vi "Create.vi"(8 "error in (no error)":errorcluster, 11 "ClientApp1 in":refnum<class "ClientApp1.lvclass">) -> (0 "error out":errorcluster, 3 "ClientApp1 out":refnum<class "ClientApp1.lvclass">)   [LabVIEW 2020, in "ClientApp1Lib.lvlib" / "ClientApp1.lvclass"]
uses:
  ClientApp1.lvclass
  C:/Users/dzoni/Documents/NJ/Playground/LV/Remote/ClientBase/ClientBase.lvclass
  ClientBase/ClientBase.lvclass
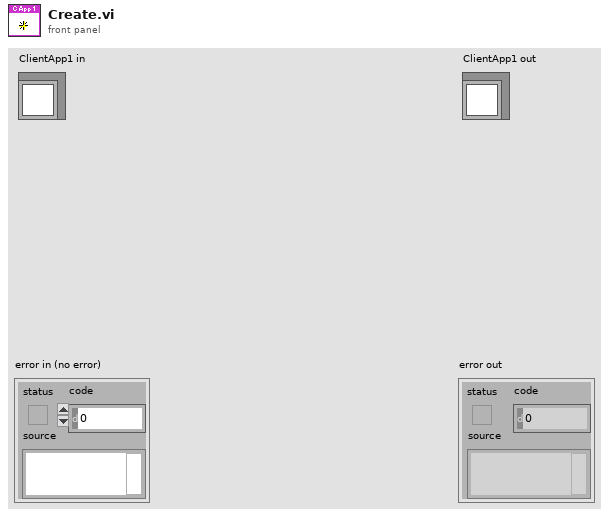
[diagram p1: front panel]
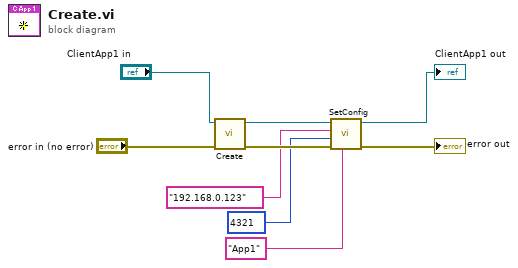
[diagram p0: block diagram]
diagram:
  n1 = call-parent "Create.vi"("error in (no error)"="error in (no error)", "ClientBase in"="ClientApp1 in") -> ("error out"=w5:errorcluster, "ClientBase out"=w7:refnum<class "ClientApp1.lvclass">)  [unwired: 8 in]
  n2 = call "SetConfig.vi"("ID"="App1", "error in (no error)"=w5, "Port"=u16 4321, "Address"="192.168.0.123", "ClientBase in"=w7) -> ("error out"=→"error out":errorcluster, "ClientBase out"=→"ClientApp1 out":refnum<class "ClientApp1.lvclass">)  [unwired: 5 in]
